vi "Populate Array Channel.vi"(8 "error in (no error)":errorcluster, 10 "Elements":T2[](array[typedef]), 11 "Array Refnum In":T1 format="%.0x") -> (0 "error out":errorcluster, 2 "Channel Refnums":T1[](array[typedef]) format="%.0x", 3 "Array Refnum Out":T1 format="%.0x")   [LabVIEW 2020, in "Instrument Addon Scripting API.lvlib"]
uses:
  Instrument Addon Scripting API.lvlib
  <vilib>/NI VeriStand/Custom Device API/Custom Device Item Ref.ctl
  TypeDefs/Array Element.ctl
  <vilib>/NI VeriStand/Custom Device API/Custom Device Channel.ctl
  <vilib>/NI VeriStand/Custom Device API/Custom Device Channel Type.ctl
  Shared Directory/Constants.vi
  <vilib>/NI VeriStand/Custom Device API/Custom Device API.lvlib
  Shared Directory/Instrument Addon Shared.lvlib
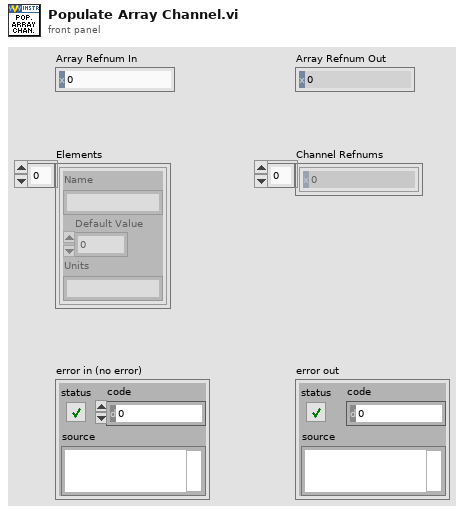
[diagram p1: front panel]
types:
  T1 = typedef "Custom Device API.lvlib/Custom Device Item Ref.ctl" = u64
  T2 = typedef "Instrument Addon Scripting API.lvlib/Array Element.ctl" = cluster{"Name":string, "Default Value":dbl, "Units":string}
  T3 = typedef "Custom Device API.lvlib/Custom Device Channel.ctl" = cluster{"Type":T4, "Units":string, "Default Value":dbl, "Faultable":bool, "Scalable":bool}
  T4 = typedef "Custom Device API.lvlib/Custom Device Channel Type.ctl" = enum16{"Input", "Output"}
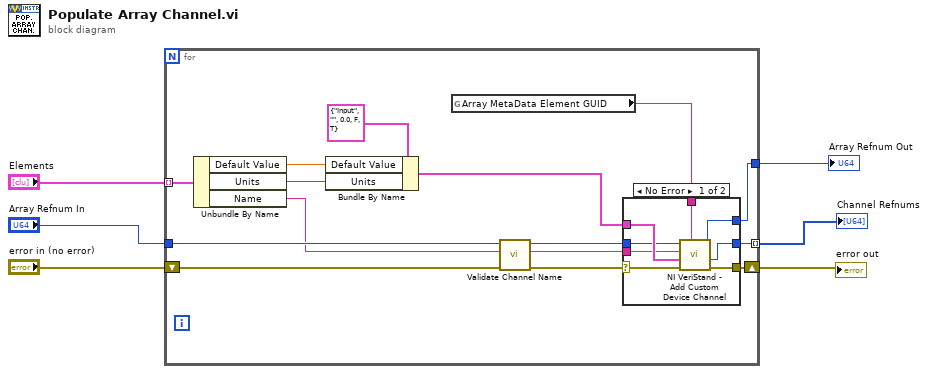
[diagram p0: block diagram]
diagram:
  n1 = for {
    shift-right: [w21] -> w6
    shift-left: "error in (no error)" -> [w7]
    tunnel: "Elements" -> [w16] mode=indexing
    tunnel: "Array Refnum In" -> [w9]
    tunnel: [w18] -> w2 mode=indexing
    tunnel: [w13] -> w1
    n2 = Unbundle By Name(w16) -> ("Default Value"=w15:dbl, "Units"=w14:string, "Name"=w8:string)
    n3 = Bundle By Name(cluster=T3 {"Type"=enum."Input", "Units"="", "Default Value"=0.0, "Faultable"=FALSE, "Scalable"=TRUE} ("Channel"), "Default Value"=w15, "Units"=w14) -> (w19:T3)
    n4 = global read "Constants.vi" "Array MetaData Element GUID"() -> (w17:string)
    n5 = call "Validate Channel Name.vi"("error in (no error)"=w7, "Name In"=w8, "Refnum In"=w9) -> ("error out"=w12:errorcluster, "Name Out"=w11:string, "Refnum Out"=w10:T1)  [unwired: 6 in]
    n6 = case shown="No Error" w12 {
      selector: w12 -> [w22 w30]
      tunnel: [w29 w30] -> w21
      tunnel: w19 -> [w28 _]
      tunnel: [w24 _] -> w18
      tunnel: w17 -> [w27 _]
      tunnel: w10 -> [w26 w31]
      tunnel: w11 -> [w25 _]
      tunnel: [w23 w31] -> w13
      frame No Error {
        n7 = call <vilib>:"NI VeriStand - Add Custom Device Channel.vi"("GUID (Default Channel)"=w27, "error in (no error)"=w22, "Channel"=w28, "Channel Name"=w25, "Parent Ref in"=w26) -> ("error out"=w29:errorcluster, "Channel Ref"=w24:T1, "Parent Ref out"=w23:T1)  [unwired: 3 in, 1 out]
      }
      frame Error {
      }
    }
  }
  "error out" <- w6
  "Channel Refnums" <- w2
  "Array Refnum Out" <- w1
